vi "z_stack_waveform_slander.vi"(4 "Z stack backward":cluster{"采样率":dbl, "采样数":dbl}={"采样率"=50000.0, "采样数"=7000.0}, 6 "Z stack acquisition":cluster{"采样率":dbl, "采样数":dbl}={"采样率"=50000.0, "采样数"=13000.0}, 7 "Steps per Volume":dbl=25.0, 9 "Backward Time (s)":dbl=0.14, 10 "SPECIFIC scan volt":dbl=5.0, 11 "Aquisition Time (s)":dbl=0.26) -> (3 "WaveformOut":waveform(dbl))   [LabVIEW 2018]
uses:
  <vilib>/Waveform/WDTOps.llb/WDT Append Waveforms DBL.vi
  <vilib>/measure/NI_MABase.lvlib
panel:
  out "Waveform Graph":waveform(dbl)(graph)
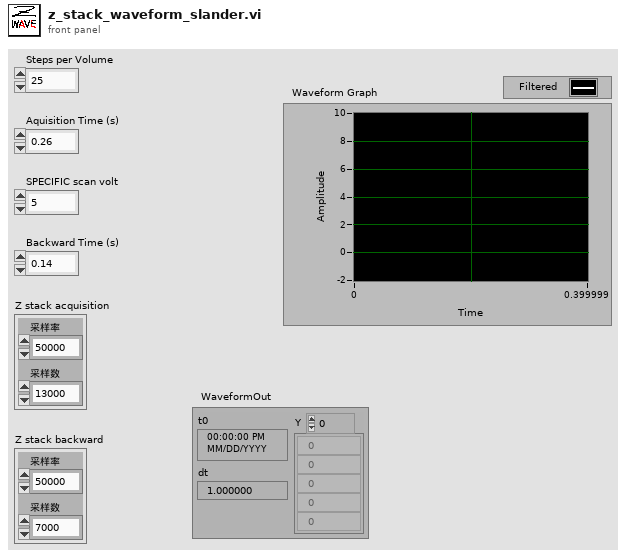
[diagram p1: front panel]
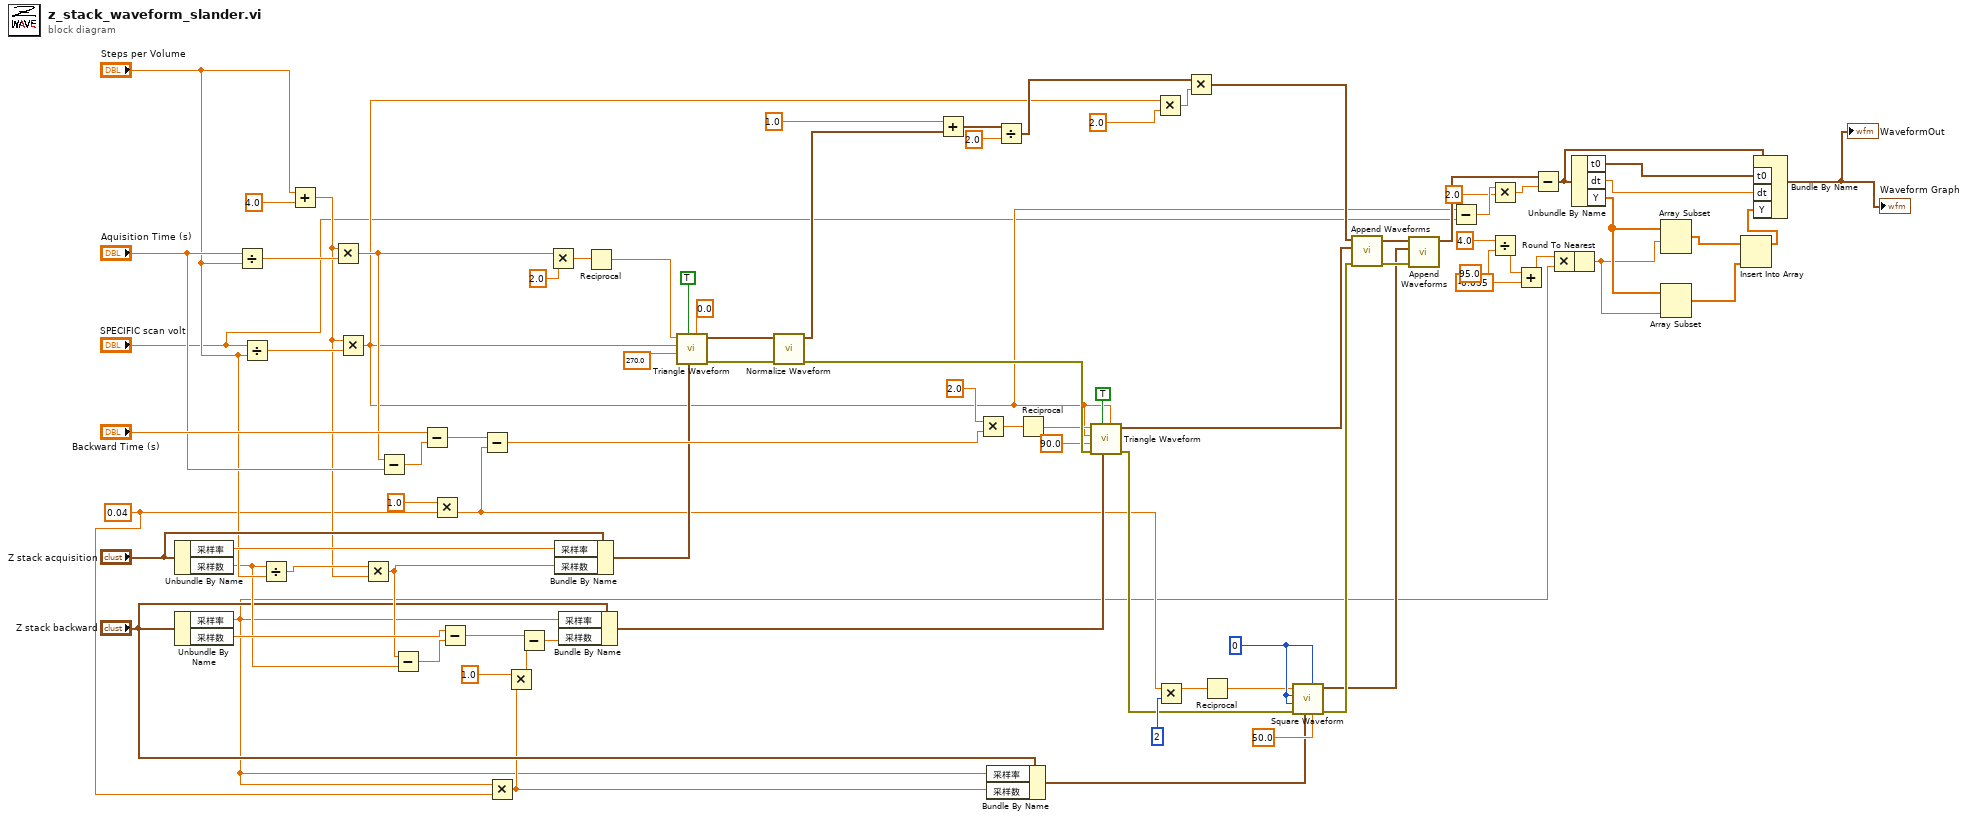
[diagram p0: block diagram]
diagram:
  w39 = 0
  w31 = 0.04
  n1 = Unbundle By Name("Z stack acquisition") -> ("采样率"=w52:dbl, "采样数"=w41:dbl)
  n2 = Unbundle By Name("Z stack backward") -> ("采样率"=w10:dbl, "采样数"=w43:dbl)
  n3 = Divide(x="Aquisition Time (s)", y="Steps per Volume") -> (x/y=w63:dbl)
  n4 = Divide(x="SPECIFIC scan volt", y="Steps per Volume") -> (x/y=w61:dbl)
  n5 = Divide(x=w41, y="Steps per Volume") -> (x/y=w49:dbl)
  n6 = Add(x="Steps per Volume", y=4.0) -> (x+y=w48:dbl)
  n7 = Multiply(x=w48, y=w63) -> (x*y=w57:dbl)
  n8 = Multiply(x=w48, y=w61) -> (x*y=w20:dbl)
  n9 = Multiply(x=w49, y=w48) -> (x*y=w40:dbl)
  n10 = Subtract(x=w57, y="Aquisition Time (s)") -> (x-y=w59:dbl)
  n11 = Subtract(x=w40, y=w41) -> (x-y=w42:dbl)
  n12 = Subtract(x="Backward Time (s)", y=w59) -> (x-y=w56:dbl)
  n13 = Multiply(x=1.0, y=w31) -> (x*y=w28:dbl)
  n14 = Subtract(x=w43, y=w42) -> (x-y=w44:dbl)
  n15 = Subtract(x=w56, y=w28) -> (x-y=w55:dbl)
  n16 = Multiply(x=w10, y=w31) -> (x*y=w30:dbl)
  n17 = Multiply(x=1.0, y=w30) -> (x*y=w26:dbl)
  n18 = Subtract(x=w44, y=w26) -> (x-y=w45:dbl)
  n19 = Multiply(x=w57, y=2.0) -> (x*y=w68:dbl)
  n20 = Bundle By Name(cluster="Z stack acquisition", "采样率"=w52, "采样数"=w40) -> (w51:cluster{"采样率":dbl, "采样数":dbl})
  n21 = Bundle By Name(cluster="Z stack backward", "采样率"=w10, "采样数"=w45) -> (w46:cluster{"采样率":dbl, "采样数":dbl})
  n22 = Reciprocal(x=w68) -> (1/x=w69:dbl)
  n23 = call <vilib>:"Triangle Waveform.vi"("offset"=0.0, "sampling info"=w51, "reset signal"=TRUE, "phase"=270.0, "amplitude"=w20, "frequency"=w69) -> ("error out"=w73:errorcluster, "signal out"=w66:waveform(dbl))  [unwired: 4 in]
  n24 = call <vilib>:"Normalize Waveform.vi"("error in (no error)"=w73, "waveform in"=w66) -> ("error out"=w84:errorcluster, "normalized waveform"=w74:waveform(dbl))  [unwired: 6 in, 2 out]
  n25 = Add(x=1.0 ("offset"), y=w74) -> (x+y=w76:waveform(dbl))
  n26 = Multiply(x=2.0 ("y"), y=w55) -> (x*y=w81:dbl)
  n27 = Bundle By Name(cluster="Z stack backward", "采样率"=w10, "采样数"=w30) -> (w29:cluster{"采样率":dbl, "采样数":dbl})
  n28 = Divide(x=w76, y=2.0 ("offset")) -> (x/y=w64:waveform(dbl))
  n29 = Reciprocal(x=w81) -> (1/x=w82:dbl)
  n30 = call <vilib>:"Triangle Waveform.vi"("offset"=w20, "sampling info"=w46, "reset signal"=TRUE, "error in (no error)"=w84, "phase"=90.0, "amplitude"=w20, "frequency"=w82) -> ("error out"=w35:errorcluster, "signal out"=w65:waveform(dbl))  [unwired: 3 in]
  n31 = Multiply(x=w20, y=2.0) -> (x*y=w78:dbl)
  n32 = Multiply(x=w28, y=2) -> (x*y=w37:dbl)
  n33 = Multiply(x=w64, y=w78) -> (x*y=w23:waveform(dbl))
  n34 = Reciprocal(x=w37) -> (1/x=w38:dbl)
  n35 = call <vilib>:"Square Waveform.vi"("duty cycle (%)"=50.0, "offset"=w39, "sampling info"=w29, "error in (no error)"=w35, "phase"=w39, "amplitude"=w39, "frequency"=w38) -> ("error out"=w34:errorcluster, "signal out"=w24:waveform(dbl))  [unwired: 3 in]
  n36 = call-poly <vilib>:"Append Waveforms.vi"("error in (no error)"=w34, "waveform B"=w65, "waveform A"=w23) -> ("error out"=w53:errorcluster, "waveform out"=w54:waveform(dbl))  [unwired: 7 in]
  n37 = call-poly <vilib>:"Append Waveforms.vi"("error in (no error)"=w53, "waveform B"=w24, "waveform A"=w54) -> ("waveform out"=w22:waveform(dbl))  [unwired: 7 in, 1 out]
  n38 = Subtract(x=w20, y="SPECIFIC scan volt") -> (x-y=w21:dbl)
  n39 = Multiply(x=w21, y=2.0) -> (x*y=w18:dbl)
  n40 = Divide(x=4.0, y=95.0) -> (x/y=w2:dbl)
  n41 = Add(x=w2, y=-0.035) -> (x+y=w3:dbl)
  n42 = Subtract(x=w22, y=w18) -> (x-y=w13:waveform(dbl))
  n43 = Multiply(x=w3, y=w10) -> (x*y=w7:dbl)
  n44 = Round To Nearest(number=w7) -> (nearest integer value=w4:dbl)
  n45 = Unbundle By Name(w13) -> ("t0"=w15:timestamp, "dt"=w14:dbl, "Y"=w8:dbl[])
  n46 = Array Subset(array=w8, index=w4) -> (w9:dbl[])  [unwired: 1 in]
  n47 = Array Subset(array=w8, length=w4) -> (w6:dbl[])  [unwired: 1 in]
  n48 = Insert Into Array(array=w9, new element=w6) -> (w5:dbl[])  [unwired: 1 in]
  n49 = Bundle By Name(cluster=w13, "t0"=w15, "dt"=w14, "Y"=w5) -> (→"WaveformOut" →"Waveform Graph":waveform(dbl))
